vi "Tosca-Init Params.vi"(0 "Tosca":refnum<class "Parameters.lvclass">, 7 "FSM.Graph":refnum<class "FSM.Graph.lvclass">, 11 "error in (no error)":errorcluster) -> (4 "Tosca Out":refnum<class "Parameters.lvclass">, 8 "FSM.Graph Out":refnum<class "FSM.Graph.lvclass">, 15 "error out":errorcluster)   [LabVIEW 2020]
uses:
  Classes/Parameters/Parameters.lvclass
  FSM Graph VIs/LV Source/Classes/FSM.Graph/FSM.Graph.lvclass
  Classes/Parameters/Parameters.lvclass/Parameters.ctl
  Classes/Parameters/Read Input Events.vi
  Classes/Parameters/Read Flags.vi
  Classes/Parameters/Write Input Events.vi
  Tosca-Globals.vi
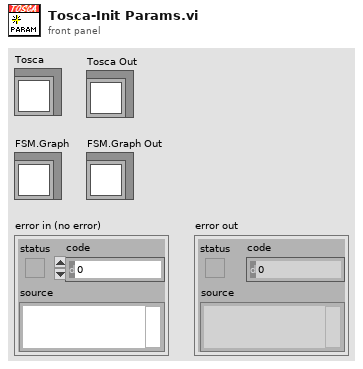
[diagram p1: front panel]
types:
  T1 = typedef "Tosca-Input Event.ctl" = cluster{"Name":string, "Criteria":T2[], "Operators":enum16{"AND", "OR"}[], "Accumulator":T4}
  T2 = typedef "Tosca-Input Criterion.ctl" = cluster{"DigInput":i32, "State":T3, "Time (ms)":i32, "Name":string}
  T3 = typedef "Logic State.ctl" = enum16{"Low", "High", "Rising", "Falling"}
  T4 = typedef "Tosca-Accumulator.ctl" = cluster{"active":bool, "N":i32, "T":dbl, "Imax":dbl, "latency":dbl}
  T5 = typedef "Tosca-Flag.ctl" = cluster{"Name":string, "Default":i32}
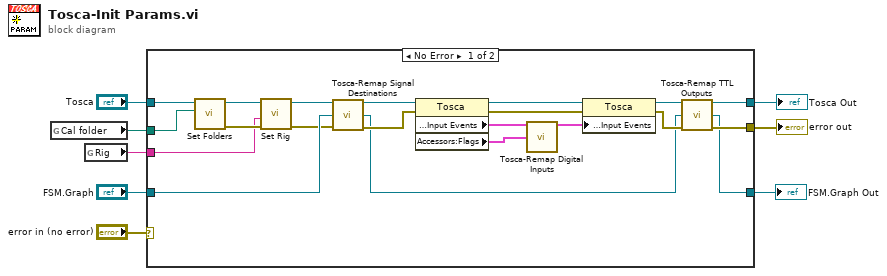
[diagram p0: block diagram]
diagram:
  n1 = global read "Tosca-Globals.vi" "Cal folder"() -> (w4:path)
  n2 = global read "Tosca-Globals.vi" "Rig"() -> (w1:string)
  n3 = case shown="No Error" "error in (no error)" {
    selector: "error in (no error)" -> [_ w31]
    tunnel: "Tosca" -> [w29 w32]
    tunnel: [w19 w32] -> w5
    tunnel: [w17 w31] -> w7
    tunnel: w4 -> [w28 _]
    tunnel: "FSM.Graph" -> [w15 w30]
    tunnel: [w16 w30] -> w2
    tunnel: w1 -> [w9 _]
    frame No Error {
      n4 = call "Set Folders.vi"("Calibration folder"=w28, "Tosca in"=w29) -> ("error out"=w11:errorcluster, "Tosca out"=w13:refnum<class "Parameters.lvclass">)  [unwired: 8 in]
      n5 = call "Set Rig.vi"("error in (no error)"=w11, "Rig"=w9, "Tosca in"=w13) -> ("error out"=w10:errorcluster, "Tosca out"=w12:refnum<class "Parameters.lvclass">)  [unwired: 7 in]
      n6 = call "Tosca-Remap Signal Destinations.vi"("Tosca"=w12, "FSM.Graph"=w15, "error in (no error)"=w10) -> ("Tosca out"=w23:refnum<class "Parameters.lvclass">, "FSM.Graph Out"=w14:refnum<class "FSM.Graph.lvclass">, "error IO"=w22:errorcluster)  [unwired: 9 in, 1 out]
      n7 = property class="Tosca"(reference=w23, error in=w22) -> (reference out=w25:refnum<class "Parameters.lvclass">, error out=w21:errorcluster, "Accessors:Input Events"=w27:T1[], "Accessors:Flags"=w26:T5[])
      n8 = call "Tosca-Remap Digital Inputs.vi"("Events In"=w27, "Flags"=w26) -> ("Events out"=w24:T1[])  [unwired: 12 in, 1 out]
      n9 = property class="Tosca"(reference=w25, error in=w21, "Accessors:Input Events"=w24) -> (reference out=w20:refnum<class "Parameters.lvclass">, error out=w18:errorcluster)
      n10 = call "Tosca-Remap TTL Outputs.vi"("Tosca"=w20, "FSM.Graph In"=w14, "error in (no error)"=w18) -> ("Tosca out"=w19:refnum<class "Parameters.lvclass">, "FSM.Graph Out"=w16:refnum<class "FSM.Graph.lvclass">, "error IO"=w17:errorcluster)  [unwired: 9 in, 1 out]
    }
    frame Error {
    }
  }
  "error out" <- w7
  "Tosca Out" <- w5
  "FSM.Graph Out" <- w2
